vi "unpack4bytes.vi"(1 "input bytes":u8[](array[numeric]) format="%x") -> (0 "number dec":u32)   [LabVIEW 2020]
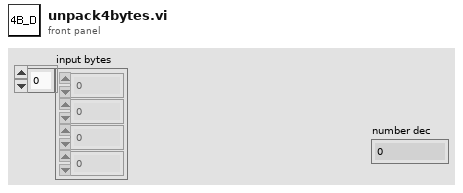
[diagram p1: front panel]
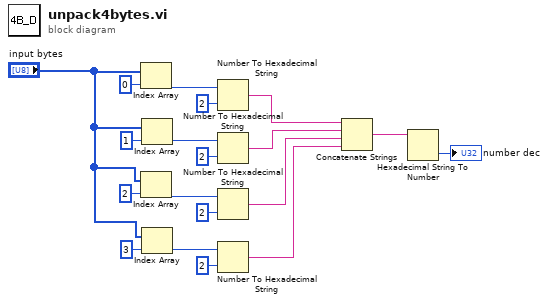
[diagram p0: block diagram]
diagram:
  n1 = Index Array(array="input bytes", index=0) -> (element=w6:u8)
  n2 = Index Array(array="input bytes", index=2) -> (element=w8:u8)
  n3 = Index Array(array="input bytes", index=1) -> (element=w9:u8)
  n4 = Index Array(array="input bytes", index=3) -> (element=w7:u8)
  n5 = Number To Hexadecimal String(1:i16 2 ("width (-)"), 2:w6) -> (0:w17:string)
  n6 = Number To Hexadecimal String(1:i16 2 ("width (-)"), 2:w9) -> (0:w16:string)
  n7 = Number To Hexadecimal String(1:i16 2 ("width (-)"), 2:w8) -> (0:w12:string)
  n8 = Number To Hexadecimal String(1:i16 2 ("width (-)"), 2:w7) -> (0:w11:string)
  n9 = Concatenate Strings(w17, w16, w12, w11) -> (w15:string)
  n10 = Hexadecimal String To Number(string=w15) -> (number=→"number dec":u32)  [unwired: 2 in, 1 out]
